vi "manual lcr control.vi"() -> ()   [LabVIEW 2018]
uses:
  <vilib>/DAQmx/write.llb/DAQmx Write (Analog DBL 1Chan 1Samp).vi
  cc3ec490-099c-4413-807a-14cffa19718a.vi
  <vilib>/DAQmx/read.llb/DAQmx Read (Analog DBL 1Chan 1Samp).vi
  <vilib>/DAQmx/create/channels.llb/DAQmx Create Channel (AO-Voltage-Basic).vi
  <vilib>/DAQmx/miscellaneous.llb/DAQmx Fill In Error Info.vi
  <vilib>/DAQmx/create/channels.llb/DAQmx Create Channel (AI-Voltage-Basic).vi
  <vilib>/ptbypt/NI_PtbyPt.lvlib
panel:
  in  "stop":bool
  out "Waveform Chart":dbl(graph)
  in  "laser tune voltage":dbl=3.79 min=0.0 max=4.0 step=0.01
  in  "sample length":i32=100
  in  "VISA resource name":refnum<visa-resource-name>="LCC25"
  in  "LCR Voltage":dbl min=0.0 max=25.0 step=0.001 format="%.3f"
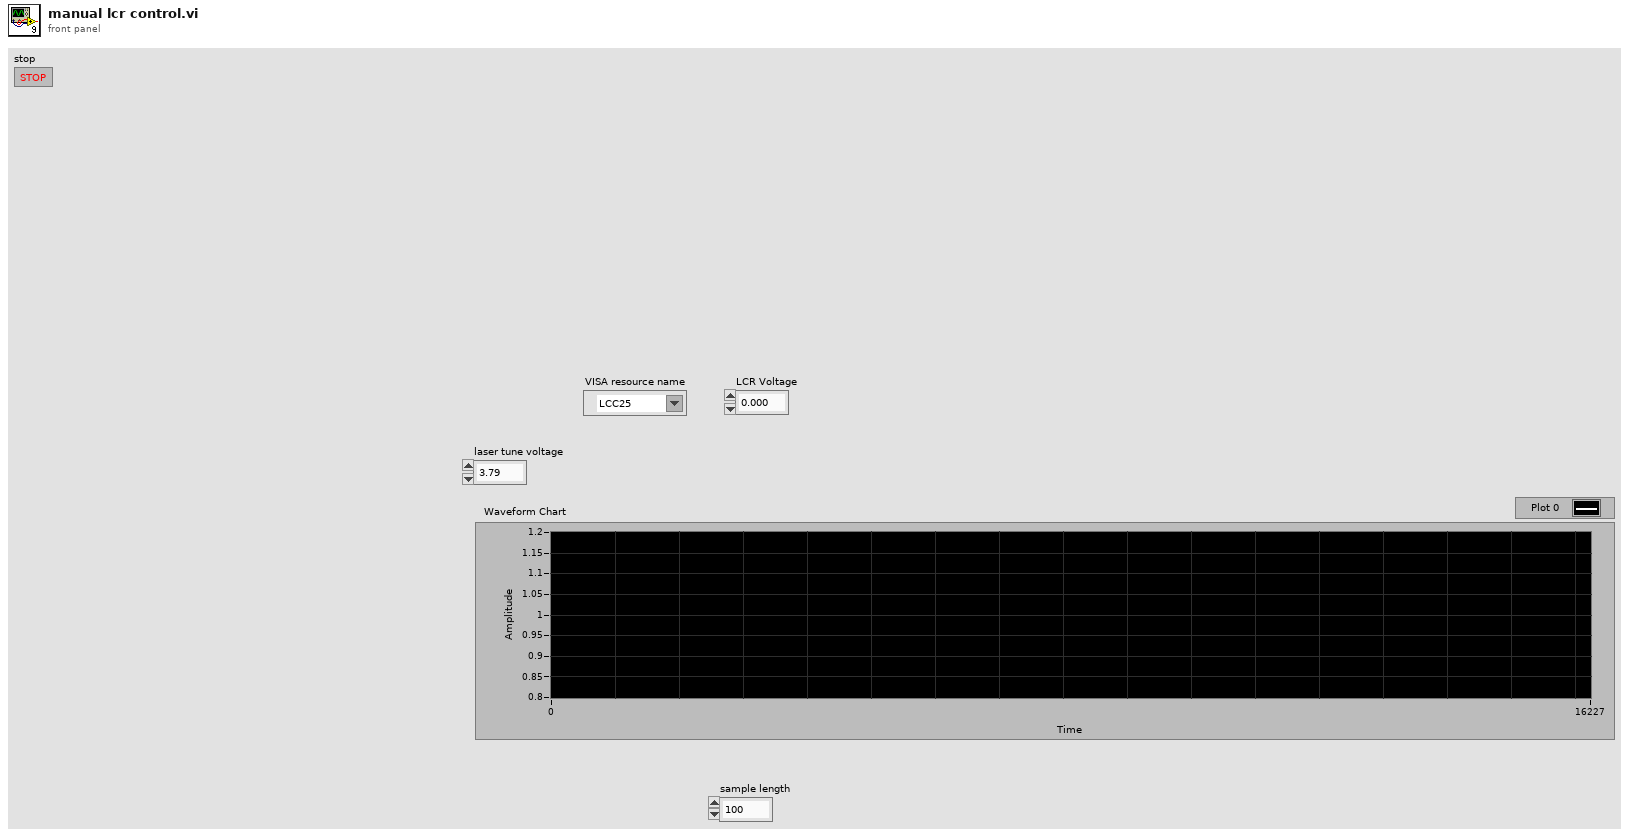
[diagram p1: front panel]
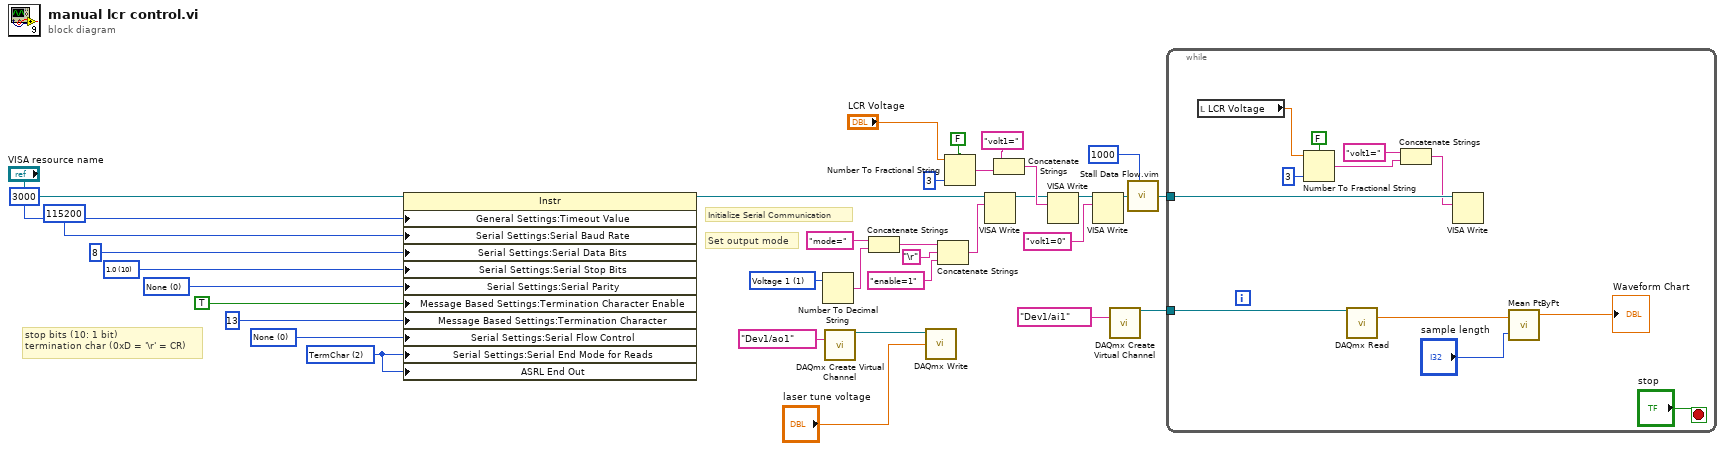
[diagram p0: block diagram]
diagram:
  w27 = u16 1 items=["Modulate", "Voltage 1", "Voltage 2"] ("Output Mode")
  w28 = u16 2 items=["None", "LastBit", "TermChar"] ("Serial Settings:Serial End Mode for Reads")
  w32 = u16 0 items=["None", "XON/XOFF", "RTS/CTS", "XON/XOFF & RTS/CTS", "DTR/DSR", "XON/XOFF & DTR/DSR"] ("flow control (0:none)")
  w30 = u16 0 items=["None", "Odd", "Even", "Mark", "Space"] ("Serial Settings:Parity")
  w34 = u16 10 items=["1.0"=10, "1.5"=15, "2.0"=20]
  # "stop bits (10: 1 bit)\ntermination char (0xD = '\\r' = CR)"
  # "Set output mode"
  # "Initialize Serial Communication"
  n1 = property class="Instr"(reference="VISA resource name", "General Settings:Timeout Value"=u32 3000 ("timeout (10sec)"), "Serial Settings:Serial Baud Rate"=u32 115200 ("baud rate (9600)115200"), "Serial Settings:Serial Data Bits"=u16 8 ("data bits (8)"), "Serial Settings:Serial Stop Bits"=w34, "Serial Settings:Serial Parity"=w30, "Message Based Settings:Termination Character Enable"=TRUE ("Enable Termination\nChar (T)"), "Message Based Settings:Termination Character"=u8 13, "Serial Settings:Serial Flow Control"=w32, "Serial Settings:Serial End Mode for Reads"=w28, "ASRL End Out"=w28) -> (reference out=w19:refnum<visa-resource-name>)  [unwired: 1 in, 1 out]
  n2 = Number To Decimal String(number=w27) -> (decimal integer string=w26:string)  [unwired: 1 in]
  n3 = call-poly <vilib>:"DAQmx Create Virtual Channel.vi"("physical channels"=tag "Dev1/ao1") -> ("task out"=w1:refnum<k21>)  [unwired: 13 in, 1 out]
  n4 = Concatenate Strings("mode=" ("string"), w26) -> (w21:string)
  n5 = call-poly <vilib>:"DAQmx Write.vi"("task/channels in"=w1, "data"="laser tune voltage") -> ()  [unwired: 11 in, 3 out]
  n6 = Concatenate Strings(w21, "\r", "enable=1" ("write buffer")) -> (w20:string)
  n7 = Number To Fractional String(use system decimal point (T)=FALSE, number="LCR Voltage", precision (6)=i16 3) -> (F-format string=w15:string)  [unwired: 1 in]
  n8 = VISA Write(VISA resource name=w19, write buffer=w20) -> (VISA resource name out=w12:refnum<visa-resource-name>)  [unwired: 1 in, 2 out]
  n9 = Concatenate Strings("volt1=" ("string"), w15) -> (w13:string)
  n10 = VISA Write(VISA resource name=w12, write buffer=w13) -> (VISA resource name out=w7:refnum<visa-resource-name>)  [unwired: 1 in, 2 out]
  n11 = VISA Write(VISA resource name=w7, write buffer="volt1=0" ("string")) -> (VISA resource name out=w8:refnum<visa-resource-name>)  [unwired: 1 in, 2 out]
  n12 = call-poly <vilib>:"DAQmx Create Virtual Channel.vi"("physical channels"=tag "Dev1/ai1") -> ("task out"=w5:refnum<k21>)  [unwired: 13 in, 1 out]
  n13 = call "Stall Data Flow.vim"("value in"=w8, "milliseconds to wait"=u32 1000) -> ("value out"=w3:refnum<visa-resource-name>)  [unwired: 1 out]
  n14 = while {
    tunnel: w3 -> [w43]
    tunnel: w5 -> [w41]
    stop <- "stop" stop-if-true
    n15 = local read "LCR Voltage"() -> (w36:dbl)
    n16 = Number To Fractional String(use system decimal point (T)=FALSE, number=w36, precision (6)=i16 3) -> (F-format string=w45:string)  [unwired: 1 in]
    n17 = call-poly <vilib>:"DAQmx Read.vi"("task/channels in"=w41) -> ("data"=w39:dbl)  [unwired: 12 in, 2 out]
    n18 = Concatenate Strings("volt1=" ("string"), w45) -> (w42:string)
    n19 = VISA Write(VISA resource name=w43, write buffer=w42) -> ()  [unwired: 1 in, 3 out]
    n20 = call <vilib>:"Mean PtByPt.vi"("x"=w39, "sample length"="sample length") -> ("mean"=→"Waveform Chart":dbl)  [unwired: 2 in, 1 out]
  }
